vi "ep_Magnitude Spectra Aggregation.vi"(0 "spectra":T2(array[cluster]), 1 "reset? (F)":bool, 5 "aggregation settings":T1={"interval"=1, "interval unit"=enum."Minutes", "synchronization of intervals"=enum."Not synchronized", "algorithm"=enum."Average"}, 9 "system info in":refnum<class "EP System Info.lvclass">, 11 "error in (no error)":errorcluster, 12 "data timestamp":timestamp) -> (4 "aggregated minimum values":T2(array[cluster]), 6 "aggregated avgeraged/RMS values":T2(array[cluster]), 8 "aggregated maximum values":T2(array[cluster]), 10 "system info out":refnum<class "EP System Info.lvclass">, 13 "aggregated data valid?":bool, 14 "aggregated data timestamp":timestamp, 15 "error out":errorcluster)   [LabVIEW 2014, in "NI_EP_Power Quality.lvlib"]
doc: "This VI accumulates input data. At every end of specified aggregation interval a minimum value, maximum value and average or RMS found within aggregation interval are provided on output. After this, the accumulation buffers are cleared and accumulation is automatically restarted."
uses:
  <vilib>/addons/Electrical Power/PQ/NI_EP_Power Quality.lvlib
  <vilib>/addons/Electrical Power/PQ/Common/Controls/ep_Aggregation Settings.ctl
  <vilib>/addons/Electrical Power/PQ/Common/Classes/System Info/EP System Info.lvclass
  <vilib>/addons/Electrical Power/PQ/Common/Controls/ep_Aggregation Data.ctl
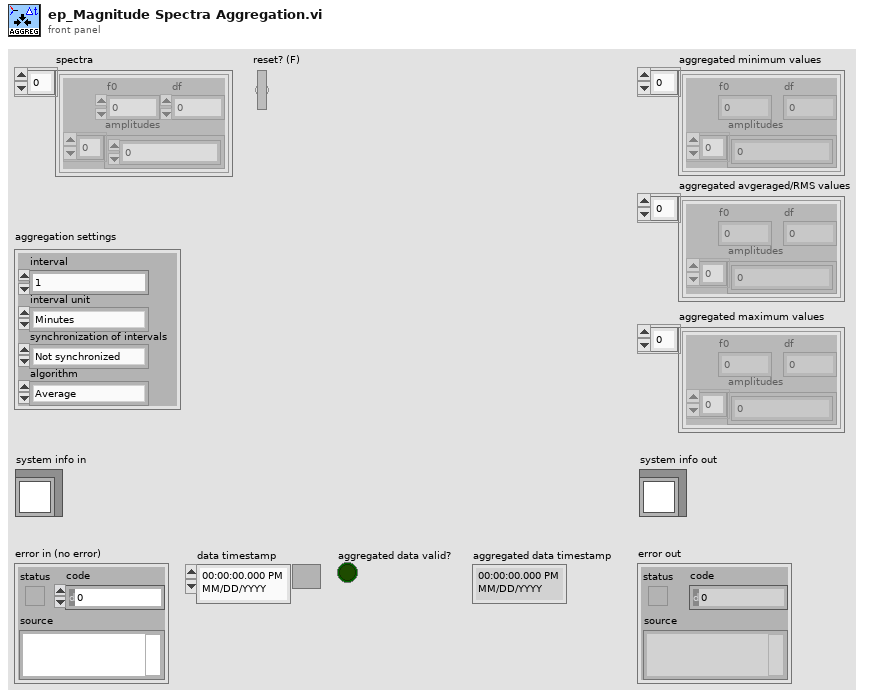
[diagram p1: front panel]
types:
  T1 = typedef "NI_EP_Power Quality.lvlib/ep_Aggregation Settings.ctl" = cluster{"interval":u32, "interval unit":enum16{"Runs", "Seconds", "Minutes", "Hours", "Days", "Weeks"}, "synchronization of intervals":enum16{"Not synchronized", "Interval rounded"}, "algorithm":enum16{"Average", "RMS"}}
  T2 = cluster{"f0":dbl, "df":dbl, "amplitudes":dbl[]}[]
  T3 = typedef "NI_EP_Power Quality.lvlib/ep_Aggregation Data.ctl" = cluster{"aggregated minimum values":dbl[], "aggregated maximum values":dbl[], "aggregated averaged/RMS values":dbl[]}
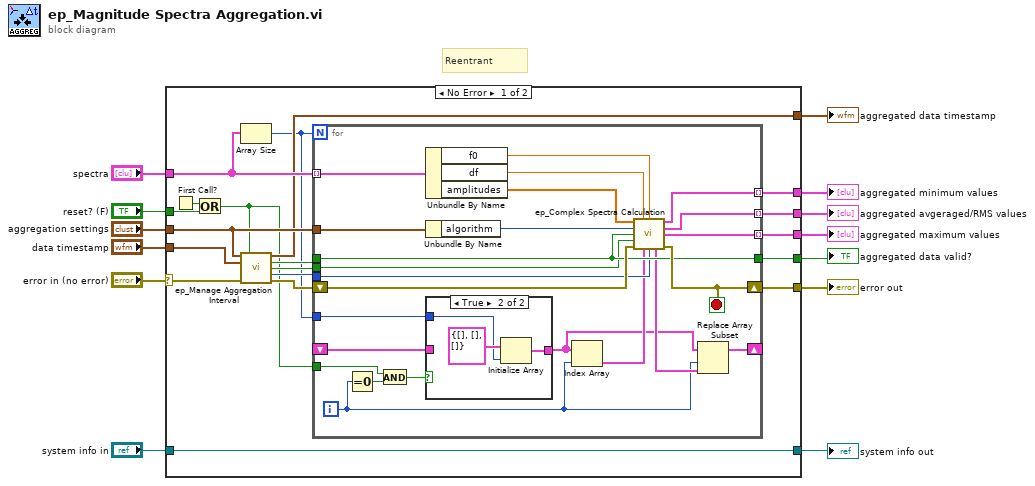
[diagram p0: block diagram]
diagram:
  # "Reentrant"
  n1 = case shown="No Error" "error in (no error)" {
    selector: "error in (no error)" -> [w27 w63]
    tunnel: [w32 w63] -> w12
    tunnel: "spectra" -> [w30 _]
    tunnel: "aggregation settings" -> [w29 _]
    tunnel: "reset? (F)" -> [w16 _]
    tunnel: "data timestamp" -> [w28 _]
    tunnel: "system info in" -> [w31 w62]
    tunnel: [w31 w62] -> w6
    tunnel: [w22 FALSE ("aggregated data valid?")] -> w5
    tunnel: [w21 _] -> w4
    tunnel: [w20 _] -> w3
    tunnel: [w19 _] -> w2
    tunnel: [w18 _] -> w1
    frame No Error {
      n2 = First Call?() -> (First Call?: T/F=w15:bool)
      n3 = Or(x=w15, y=w16) -> (x .or. y?=w14:bool)
      n4 = Array Size(array=w30) -> (size(s)=w17:i32)
      n5 = call <vilib>:"ep_Manage Aggregation Interval.vi"("aggregation settings"=w29, "restart (F)"=w14, "data time stamp"=w28, "error in (no error)"=w27) -> ("aggregated data time stamp"=w21:timestamp, "aggregated data valid?"=w24:bool, "restart aggregation?"=w25:bool, "runs"=w23:u32, "error out"=w26:errorcluster)  [unwired: 7 in]
      n6 = for {
        N: w17 -> [_]
        shift-right: [w45] -> w32
        shift-left: w26 -> [w51]
        tunnel: w30 -> [w56] mode=indexing
        tunnel: w29 -> [w54]
        shift-right: [w53] -> _
        shift-left: _ -> [w38]
        tunnel: w25 -> [w43]
        tunnel: w24 -> [w44]
        tunnel: w23 -> [w42]
        tunnel: [w44] -> w22
        tunnel: [w48] -> w20 mode=indexing
        tunnel: [w47] -> w19 mode=indexing
        tunnel: [w46] -> w18 mode=indexing
        tunnel: w17 -> [w37]
        tunnel: w14 -> [w35]
        i -> [w33]
        stop <- w45 stop-if-true
        n7 = Equal To 0?(x=w33) -> (x = 0?=w36:bool)
        n8 = And(x=w35, y=w36) -> (x .and. y?=w34:bool)
        n9 = Unbundle By Name(w56) -> ("f0"=w49:dbl, "df"=w50:dbl, "amplitudes"=w55:dbl[])
        n10 = Unbundle By Name(w54) -> ("algorithm"=w52:enum16{"Average", "RMS"})
        n11 = case shown="True" w34 {
          tunnel: [w57 w59] -> w39
          tunnel: w37 -> [_ w58]
          tunnel: w38 -> [w57 _]
          frame False {
          }
          frame True {
            n12 = Initialize Array(T3 {"aggregated minimum values"=[], "aggregated maximum values"=[], "aggregated averaged/RMS values"=[]} ("aggregated data"), w58) -> (w59:T3[])
          }
        }
        n13 = Index Array(array=w39, index=w33) -> (element=w41:T3)
        n14 = call <vilib>:"ep_Complex Spectra Calculation.vi"("data in"=w55, "df"=w50, "f0"=w49, "algorithm"=w52, "aggregated data valid? (F)"=w44, "restart aggregation? (F)"=w43, "error in (no error)"=w51, "aggregated data"=w41, "runs"=w42) -> ("aggregated minimum values"=w48:cluster{"f0":dbl, "df":dbl, "amplitudes":dbl[]}, "aggregated avgeraged/RMS values"=w47:cluster{"f0":dbl, "df":dbl, "amplitudes":dbl[]}, "aggregated maximum values"=w46:cluster{"f0":dbl, "df":dbl, "amplitudes":dbl[]}, "aggregated data"=w40:T3, "error out"=w45:errorcluster)  [unwired: 2 in]
        n15 = Replace Array Subset(array=w39, new element=w40, index=w33) -> (w53:T3[])
      }
    }
    frame Error {
    }
  }
  "error out" <- w12
  "aggregated minimum values" <- w3
  "aggregated avgeraged/RMS values" <- w2
  "aggregated maximum values" <- w1
  "aggregated data valid?" <- w5
  "aggregated data timestamp" <- w4
  "system info out" <- w6
